vi "Camera_Config.vi"(8 "error in (no error)":errorcluster, 10 "crop?":bool, 11 "DataCluster in":T1={"Core"={"Current VI Reference"=refnum, "Close Panel on Exit?"=FALSE, "Exit"=FALSE, "Initialized?"=FALSE}, "Connections"={"cDAQ"={"Task"="", "Connected"=FALSE, "Active"=FALSE, "ID"=""}, "Camera"={"Session"="", "Connected"=FALSE, "Active"=FALSE, "Placeholder"=refnum}, "PSU"={"Port"="", "Connected"=FALSE, "Active"=FALSE}, "Arduino"={"Port"="", "Connected"=FALSE, "Active"=FALSE}}, "Data Acquisition"={"Setup"={"Label"="", "Operator"="", "Notes"="", "TempGrad"=1.0, "TargetTemp"=1.0, "Sample Volume"=1.0}, "Camera"={"Image"=refnum, "Save Image"=refnum, "Image Frequency"=20, "Rectangle"={"Left"=0, "Top"=0, "Right"=0, "Bottom"=0, "Rotation"=0.0}, "Calibration"={"Top Left"={"X"=0.0, "Y"=0.0}, "Top Right"={"X"=0.0, "Y"=0.0}, "Bottom Left"={"X"=0.0, "Y"=0.0}, "Bottom Right"={"X"=0.0, "Y"=0.0}, "Fixpoint"={"X"=0.0, "Y"=0.0}, "Scan Area"=0.0, "Fixpoint Area"=0.0, "Well Pixels"=[], "Valid"=FALSE}, "FocusPos"=0, "Display Mapping"=10}, "Thermistor"={"Sample Size"=1, "Calibration"={"B0.100"=[], "R25"=[], "c"=[], "State"=[], "V_S"=5.0, "R_S"=100.0}, "Timing Mode"=14713}, "Partition"={"Data"=[], "Cell Label"="", "Cell Color"=0, "Height"=10, "Width"=16, "Grid"=[]}, "Queue"={"Size"=1, "Queue"=refnum}, "Sample Rate"=1, "Active"=FALSE, "Ready"=FALSE, "Graph Mode"=0, "Gradient Buffer"=2}, "Control"={"Sample Rate"=1, "PID gains"={"proportional gain (Kc)"=1.0, "integral time (Ti, min)"=0.01, "derivative time (Td, min)"=0.0}}, "Manual Temp Control"={"TargetTemp"=1.0, "Mode"=0, "Active"=FALSE}} {"Manual Temp Control"."Mode" items=["Cool", "Heat"]; "Manual Temp Control"."TargetTemp" min=-40.0 max=40.0 step=0.5 format="%#_g °C"; "Control"."PID gains"."derivative time (Td, min)" format="%.3f"; "Control"."PID gains"."integral time (Ti, min)" format="%.3f"; "Control"."PID gains"."proportional gain (Kc)" format="%.3f"; "Control"."Sample Rate" min=1 max=20 step=1 format="%.0f Samples/sec"; "Data Acquisition"."Gradient Buffer" min=2 max=30 step=1; "Data Acquisition"."Graph Mode" items=["Thermistor Temperature", "Camera Temperature"]; "Data Acquisition"."Thermistor"."Timing Mode" items=["Automatic"=16097, "High Resolution"=10195, "High Speed"=14712, "Best 50 Hz Rejection"=14713, "Best 60 Hz Rejection"=14714, "Custom"=10137]; "Data Acquisition"."Thermistor"."Calibration"."R_S" min=0.1 max=1000.0 format="%#_g kOhm"; "Data Acquisition"."Thermistor"."Calibration"."V_S" min=5.0 max=48.0 format="%#_g V"; "Data Acquisition"."Thermistor"."Calibration"."R25" min=0.1 max=1000.0 format="%#_g kOhm"; "Data Acquisition"."Thermistor"."Calibration"."B0.100" min=100.0 max=10000.0 format="%#_g K"; "Data Acquisition"."Thermistor"."Sample Size" min=1 max=200; "Data Acquisition"."Sample Rate" min=20 max=240 format="%.0f samples/min"; "Data Acquisition"."Queue"."Size" min=1 max=200; "Data Acquisition"."Camera"."Display Mapping" items=["Default"=10, "Most Significant Bits"=11, "Full Dynamic"=12, "Downshift"=13, "Given Range"=14, "90% Dynamic"=15, "Given Percent Range"=16]; "Data Acquisition"."Camera"."Calibration"."Fixpoint"."Y" format="%.2f"; "Data Acquisition"."Camera"."Calibration"."Fixpoint"."X" format="%.2f"; "Data Acquisition"."Camera"."Calibration"."Top Left"."Y" format="%.2f"; "Data Acquisition"."Camera"."Calibration"."Top Left"."X" format="%.2f"; "Data Acquisition"."Camera"."Calibration"."Top Right"."Y" format="%.2f"; "Data Acquisition"."Camera"."Calibration"."Top Right"."X" format="%.2f"; "Data Acquisition"."Camera"."Calibration"."Bottom Left"."Y" format="%.2f"; "Data Acquisition"."Camera"."Calibration"."Bottom Left"."X" format="%.2f"; "Data Acquisition"."Camera"."Calibration"."Bottom Right"."Y" format="%.2f"; "Data Acquisition"."Camera"."Calibration"."Bottom Right"."X" format="%.2f"; "Data Acquisition"."Camera"."Rectangle"."Rotation" min=-90.0 max=90.0 step=1.0 format="%.2f"; "Data Acquisition"."Camera"."Rectangle"."Left" scale=0.0..1024.0; "Data Acquisition"."Camera"."Rectangle"."Right" scale=0.0..1024.0; "Data Acquisition"."Camera"."Image Frequency" min=1 max=60 step=1; "Data Acquisition"."Setup"."Sample Volume" min=0.0 max=500.0 format="%#_g µL"; "Data Acquisition"."Setup"."TargetTemp" min=-40.0 max=40.0 step=0.5 format="%#_g °C"; "Data Acquisition"."Setup"."TempGrad" min=-100.0 max=100.0 step=0.1 format="%#_g °C/min"}) -> (0 "error out":errorcluster, 3 "DataCluster out":T1={"Core"={"Current VI Reference"=refnum, "Close Panel on Exit?"=FALSE, "Exit"=FALSE, "Initialized?"=FALSE}, "Connections"={"cDAQ"={"Task"="", "Connected"=FALSE, "Active"=FALSE, "ID"=""}, "Camera"={"Session"="", "Connected"=FALSE, "Active"=FALSE, "Placeholder"=refnum}, "PSU"={"Port"="", "Connected"=FALSE, "Active"=FALSE}, "Arduino"={"Port"="", "Connected"=FALSE, "Active"=FALSE}}, "Data Acquisition"={"Setup"={"Label"="", "Operator"="", "Notes"="", "TempGrad"=1.0, "TargetTemp"=1.0, "Sample Volume"=1.0}, "Camera"={"Image"=refnum, "Save Image"=refnum, "Image Frequency"=20, "Rectangle"={"Left"=0, "Top"=0, "Right"=0, "Bottom"=0, "Rotation"=0.0}, "Calibration"={"Top Left"={"X"=0.0, "Y"=0.0}, "Top Right"={"X"=0.0, "Y"=0.0}, "Bottom Left"={"X"=0.0, "Y"=0.0}, "Bottom Right"={"X"=0.0, "Y"=0.0}, "Fixpoint"={"X"=0.0, "Y"=0.0}, "Scan Area"=0.0, "Fixpoint Area"=0.0, "Well Pixels"=[], "Valid"=FALSE}, "FocusPos"=0, "Display Mapping"=10}, "Thermistor"={"Sample Size"=1, "Calibration"={"B0.100"=[], "R25"=[], "c"=[], "State"=[], "V_S"=5.0, "R_S"=100.0}, "Timing Mode"=14713}, "Partition"={"Data"=[], "Cell Label"="", "Cell Color"=0, "Height"=10, "Width"=16, "Grid"=[]}, "Queue"={"Size"=1, "Queue"=refnum}, "Sample Rate"=1, "Active"=FALSE, "Ready"=FALSE, "Graph Mode"=0, "Gradient Buffer"=2}, "Control"={"Sample Rate"=1, "PID gains"={"proportional gain (Kc)"=1.0, "integral time (Ti, min)"=0.01, "derivative time (Td, min)"=0.0}}, "Manual Temp Control"={"TargetTemp"=1.0, "Mode"=0, "Active"=FALSE}} {"Manual Temp Control"."Mode" items=["Cool", "Heat"]; "Manual Temp Control"."TargetTemp" min=-40.0 max=40.0 step=0.5 format="%#_g °C"; "Control"."PID gains"."derivative time (Td, min)" format="%.3f"; "Control"."PID gains"."integral time (Ti, min)" format="%.3f"; "Control"."PID gains"."proportional gain (Kc)" format="%.3f"; "Control"."Sample Rate" min=1 max=20 step=1 format="%.0f Samples/sec"; "Data Acquisition"."Gradient Buffer" min=2 max=30 step=1; "Data Acquisition"."Graph Mode" items=["Thermistor Temperature", "Camera Temperature"]; "Data Acquisition"."Thermistor"."Timing Mode" items=["Automatic"=16097, "High Resolution"=10195, "High Speed"=14712, "Best 50 Hz Rejection"=14713, "Best 60 Hz Rejection"=14714, "Custom"=10137]; "Data Acquisition"."Thermistor"."Calibration"."R_S" min=0.1 max=1000.0 format="%#_g kOhm"; "Data Acquisition"."Thermistor"."Calibration"."V_S" min=5.0 max=48.0 format="%#_g V"; "Data Acquisition"."Thermistor"."Calibration"."R25" min=0.1 max=1000.0 format="%#_g kOhm"; "Data Acquisition"."Thermistor"."Calibration"."B0.100" min=100.0 max=10000.0 format="%#_g K"; "Data Acquisition"."Thermistor"."Sample Size" min=1 max=200; "Data Acquisition"."Sample Rate" min=20 max=240 format="%.0f samples/min"; "Data Acquisition"."Queue"."Size" min=1 max=200; "Data Acquisition"."Camera"."Display Mapping" items=["Default"=10, "Most Significant Bits"=11, "Full Dynamic"=12, "Downshift"=13, "Given Range"=14, "90% Dynamic"=15, "Given Percent Range"=16]; "Data Acquisition"."Camera"."Calibration"."Fixpoint"."Y" format="%.2f"; "Data Acquisition"."Camera"."Calibration"."Fixpoint"."X" format="%.2f"; "Data Acquisition"."Camera"."Calibration"."Top Left"."Y" format="%.2f"; "Data Acquisition"."Camera"."Calibration"."Top Left"."X" format="%.2f"; "Data Acquisition"."Camera"."Calibration"."Top Right"."Y" format="%.2f"; "Data Acquisition"."Camera"."Calibration"."Top Right"."X" format="%.2f"; "Data Acquisition"."Camera"."Calibration"."Bottom Left"."Y" format="%.2f"; "Data Acquisition"."Camera"."Calibration"."Bottom Left"."X" format="%.2f"; "Data Acquisition"."Camera"."Calibration"."Bottom Right"."Y" format="%.2f"; "Data Acquisition"."Camera"."Calibration"."Bottom Right"."X" format="%.2f"; "Data Acquisition"."Camera"."Rectangle"."Rotation" min=-90.0 max=90.0 step=1.0 format="%.2f"; "Data Acquisition"."Camera"."Rectangle"."Left" scale=0.0..1024.0; "Data Acquisition"."Camera"."Rectangle"."Right" scale=0.0..1024.0; "Data Acquisition"."Camera"."Image Frequency" min=1 max=60 step=1; "Data Acquisition"."Setup"."Sample Volume" min=0.0 max=500.0 format="%#_g µL"; "Data Acquisition"."Setup"."TargetTemp" min=-40.0 max=40.0 step=0.5 format="%#_g °C"; "Data Acquisition"."Setup"."TempGrad" min=-100.0 max=100.0 step=0.1 format="%#_g °C/min"})   [LabVIEW 2022 SP3]
uses:
  DataCluster.ctl
  <vilib>/userdefined/High Color/IMAQdx.ctl
  <vilib>/vision/Image Controls.llb/IMAQ Image.ctl
  <vilib>/vision/driver/IMAQdx.llb/IMAQdx Acquisition Mode.ctl
  <vilib>/vision/driver/NI_Vision_Acquisition_Software.lvlib
  <resource>/objmgr/imaqdx.rc
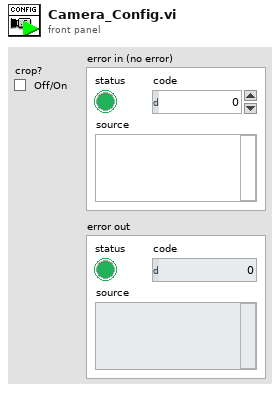
[diagram p1: front panel]
types:
  T1 = typedef "DataCluster.ctl" = cluster{"Core":cluster{"Current VI Reference":refnum<vi>, "Close Panel on Exit?":bool, "Exit":bool, "Initialized?":bool}, "Connections":cluster{"cDAQ":cluster{"Task":refnum<k21>, "Connected":bool, "Active":bool, "ID":string}, "Camera":cluster{"Session":T2, "Connected":bool, "Active":bool, "Placeholder":T3}, "PSU":cluster{"Port":refnum<visa-resource-name>, "Connected":bool, "Active":bool}, "Arduino":cluster{"Port":refnum<visa-resource-name>, "Connected":bool, "Active":bool}}, "Data Acquisition":cluster{"Setup":cluster{"Label":string, "Operator":string, "Notes":string, "TempGrad":dbl, "TargetTemp":dbl, "Sample Volume":dbl}, "Camera":cluster{"Image":T3, "Save Image":T3, "Image Frequency":i32, "Rectangle":T4, "Calibration":cluster{"Top Left":T5, "Top Right":T5, "Bottom Left":T5, "Bottom Right":T5, "Fixpoint":T5, "Scan Area":dbl, "Fixpoint Area":dbl, "Well Pixels":cluster{"X":i32, "Y":i32}[][], "Valid":bool}, "FocusPos":u32, "Display Mapping":u32}, "Thermistor":cluster{"Sample Size":i32, "Calibration":cluster{"B0.100":dbl[], "R25":dbl[], "c":dbl[][], "State":bool[], "V_S":dbl, "R_S":dbl}, "Timing Mode":i32}, "Partition":cluster{"Data":string[][], "Cell Label":string, "Cell Color":u32, "Height":i32, "Width":i32, "Grid":string[][]}, "Queue":cluster{"Size":i32, "Queue":refnum<queue>}, "Sample Rate":i32, "Active":bool, "Ready":bool, "Graph Mode":u16, "Gradient Buffer":i32}, "Control":cluster{"Sample Rate":i32, "PID gains":cluster{"proportional gain (Kc)":dbl, "integral time (Ti, min)":dbl, "derivative time (Td, min)":dbl}}, "Manual Temp Control":cluster{"TargetTemp":dbl, "Mode":u16, "Active":bool}}
  T2 = typedef "IMAQdx.ctl" = refnum<k21>
  T3 = typedef "IMAQ Image.ctl" = refnum<image>
  T4 = typedef "IMAQ Rectangle" = cluster{"Left":i32, "Top":i32, "Right":i32, "Bottom":i32, "Rotation":dbl}
  T5 = typedef "IMAQ Point" = cluster{"X":sgl, "Y":sgl}
  T6 = typedef "NI_Vision_Acquisition_Software.lvlib/IMAQdx Acquisition Mode.ctl" = enum32{"One Shot", "Continuous"}
  T7 = typedef "Image Type" = u32
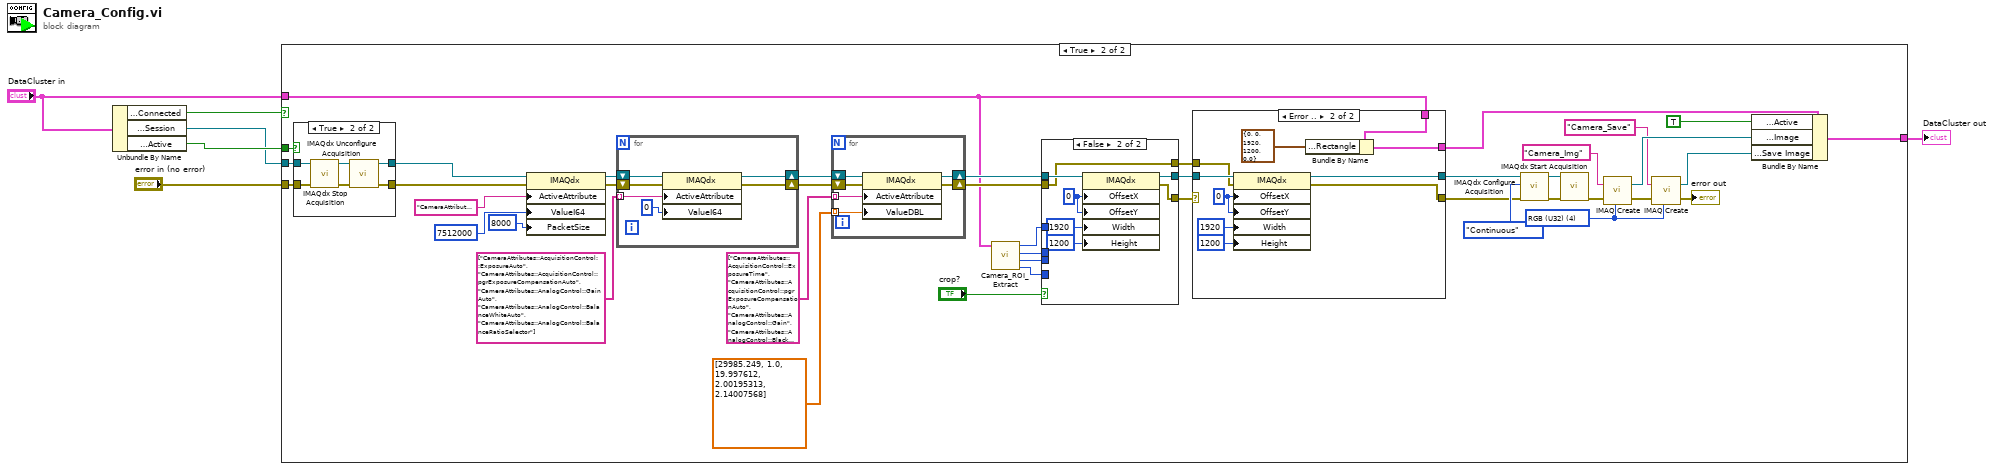
[diagram p0: block diagram]
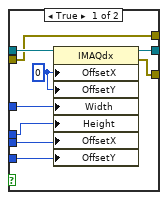
[diagram p5: hidden frame]
diagram:
  n1 = Unbundle By Name("DataCluster in") -> ("Connections.Camera.Connected"=w1:bool, "Connections.Camera.Session"=w2:T2, "Connections.Camera.Active"=w4:bool)
  n2 = case shown="True" w1 {
    tunnel: [w7 w49] -> w6
    tunnel: "DataCluster in" -> [w7 w10]
    tunnel: w4 -> [_ w23]
    tunnel: "error in (no error)" -> [_ w22]
    tunnel: w2 -> [_ w21]
    frame False {
    }
    frame True {
      w27 = T7 4 items=["Grayscale (U8)", "Grayscale (I16)", "Grayscale (SGL)", "Complex (CSG)", "RGB (U32)", "HSL (U32)", "RGB (U64)", "Grayscale (U16)"] ("Image Type")
      n3 = case shown="True" w23 {
        tunnel: w22 -> [w63 w68]
        tunnel: w21 -> [w64 w67]
        tunnel: [w64 w66] -> w20
        tunnel: [w63 w65] -> w19
        frame False {
        }
        frame True {
          n4 = call <vilib>:"IMAQdx Stop Acquisition.vi"("error in"=w68, "Session In"=w67) -> ("error out"=w69:errorcluster, "Session Out"=w70:T2)  [unwired: 8 in]
          n5 = call <vilib>:"IMAQdx Unconfigure Acquisition.vi"("error in"=w69, "Session In"=w70) -> ("error out"=w65:errorcluster, "Session Out"=w66:T2)  [unwired: 8 in]
        }
      }
      n6 = property class="IMAQdx"(reference=w20, error in=w19, "ActiveAttribute"="CameraAttributes::DeviceControl::DeviceLinkThroughputLimit", "ValueI64"=i64 7512000, "PacketSize"=u32 8000) -> (reference out=w32:T2, error out=w33:errorcluster)
      n7 = for {
        tunnel: string[] ["CameraAttributes::AcquisitionControl::ExposureAuto", "CameraAttributes::AcquisitionControl::pgrExposureCompensationAuto", "CameraAttributes::AnalogControl::GainAuto", "CameraAttributes::AnalogControl::BalanceWhiteAuto", "CameraAttributes::AnalogControl::BalanceRatioSelector"] -> [w97] mode=indexing
        shift-right: [w94] -> w29
        shift-left: w32 -> [w95]
        shift-right: [w93] -> w28
        shift-left: w33 -> [w96]
        n8 = property class="IMAQdx"(reference=w95, error in=w96, "ActiveAttribute"=w97, "ValueI64"=i64 0) -> (reference out=w94:T2, error out=w93:errorcluster)
      }
      n9 = for {
        shift-right: [w90] -> w26
        shift-left: w29 -> [w92]
        shift-right: [w87] -> w25
        shift-left: w28 -> [w91]
        tunnel: string[] ["CameraAttributes::AcquisitionControl::ExposureTime", "CameraAttributes::AcquisitionControl::pgrExposureCompensationAuto", "CameraAttributes::AnalogControl::Gain", "CameraAttributes::AnalogControl::BlackLevel", "CameraAttributes::AnalogControl::BalanceRatio"] -> [w89] mode=indexing
        tunnel: dbl[] [29985.249, 1.0, 19.997612, 2.00195313, 2.14007568] -> [w88] mode=indexing
        n10 = property class="IMAQdx"(reference=w92, error in=w91, "ActiveAttribute"=w89, "ValueDBL"=w88) -> (reference out=w90:T2, error out=w87:errorcluster)
      }
      n11 = call "Camera_ROI_Extract.vi"("input cluster"=w10) -> ("Offset Y"=w15:u32, "Offset X"=w16:u32, "Height"=w17:u32, "Width"=w18:u32)  [unwired: 7 in]
      n12 = case shown="False" "crop?" {
        tunnel: w26 -> [w79 w86]
        tunnel: w25 -> [w71 w80]
        tunnel: [w78 w85] -> w13
        tunnel: [w77 w84] -> w14
        tunnel: w18 -> [w75 _]
        tunnel: w17 -> [w74 _]
        tunnel: w16 -> [w73 _]
        tunnel: w15 -> [w72 _]
        tunnel: [w71 w80] -> w8
        frame True {
          w76 = u32 0 ("OffsetX")
          n13 = property class="IMAQdx"(reference=w79, "OffsetX"=w76, "OffsetY"=w76, "Width"=w75, "Height"=w74, "OffsetX"=w73, "OffsetY"=w72) -> (reference out=w78:T2, error out=w77:errorcluster)  [unwired: 1 in]
        }
        frame False {
          w83 = u32 0 ("OffsetX")
          n14 = property class="IMAQdx"(reference=w86, "OffsetX"=w83, "OffsetY"=w83, "Width"=u32 1920, "Height"=u32 1200) -> (reference out=w85:T2, error out=w84:errorcluster)  [unwired: 1 in]
        }
      }
      n15 = case shown="Error .." w14 {
        selector: w14 -> [w51 _]
        tunnel: w13 -> [w52 w59]
        tunnel: [w52 w58] -> w12
        tunnel: [w51 w57] -> w11
        tunnel: w10 -> [w50 w56]
        tunnel: [w50 w54] -> w9
        tunnel: w8 -> [_ w53]
        frame No Error {
        }
        frame Error {
          w60 = u32 0 ("OffsetX")
          n16 = property class="IMAQdx"(reference=w59, error in=w53, "OffsetX"=w60, "OffsetY"=w60, "Width"=u32 1920, "Height"=u32 1200) -> (reference out=w58:T2, error out=w57:errorcluster)
          n17 = Bundle By Name(cluster=w56, "Data Acquisition.Camera.Rectangle"=T4 {"Left"=0, "Top"=0, "Right"=1920, "Bottom"=1200, "Rotation"=0.0}) -> (w54:T1)
        }
      }
      n18 = call <vilib>:"IMAQdx Configure Acquisition.vi"("error in"=w11, "Continuous?"=IMAQdx_Acquisition_Mode."Continuous", "Session In"=w12) -> ("error out"=w45:errorcluster, "Session Out"=w46:T2)  [unwired: 7 in]
      n19 = call <vilib>:"IMAQdx Start Acquisition.vi"("error in"=w45, "Session In"=w46) -> ("error out"=w42:errorcluster)  [unwired: 8 in, 1 out]
      n20 = call "IMAQ Create"("Image Name"="Camera_Img", "Image Type"=w27, "error in (no error)"=w42) -> ("New Image"=w43:T3, "error out"=w40:errorcluster)  [unwired: 2 in]
      n21 = call "IMAQ Create"("Image Name"="Camera_Save", "Image Type"=w27, "error in (no error)"=w40) -> ("New Image"=w38:T3, "error out"=→"error out":errorcluster)  [unwired: 2 in]
      n22 = Bundle By Name(cluster=w9, "Connections.Camera.Active"=TRUE, "Data Acquisition.Camera.Image"=w43, "Data Acquisition.Camera.Save Image"=w38) -> (w49:T1)
    }
  }
  "DataCluster out" <- w6
